vi "Read PublicEvents.vi"(8 "error in (no error)":errorcluster, 11 "SMOFacade in":refnum<class "SMOFacade.lvclass">) -> (0 "error out":errorcluster, 2 "SMO Base Events":T1, 3 "SMOFacade out":refnum<class "SMOFacade.lvclass">)   [LabVIEW 2013, in "SMOFacade.lvclass"]
uses:
  SMOFacade.lvclass
  SMO/Typedefs/Public Events.ctl
  SMO/Typedefs/SMOState --Enum.ctl
  SMO/Typedefs/Reserve State--Enum.ctl
  SMOFacade.lvclass/SMOFacade.ctl
  PublicEvents/PublicEvents.lvclass/PublicEvents.ctl
  PublicEvents/PublicEvents.lvclass
  SMO/SMO.lvclass
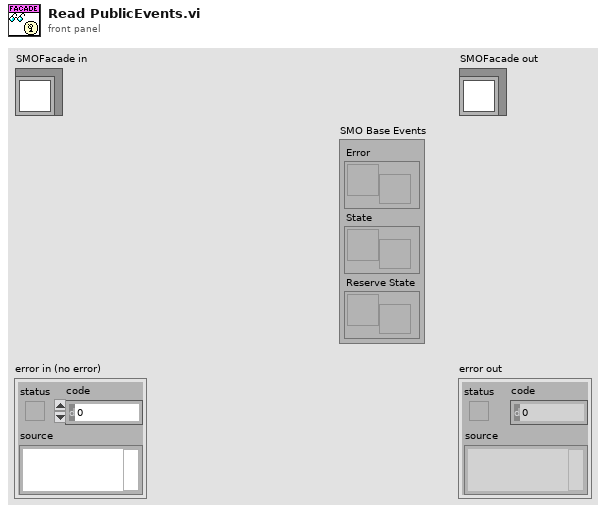
[diagram p1: front panel]
types:
  T1 = typedef "SMO.lvclass/Public Events.ctl" = cluster{"Error":refnum<user-event>, "State":refnum<user-event>, "Reserve State":refnum<user-event>}
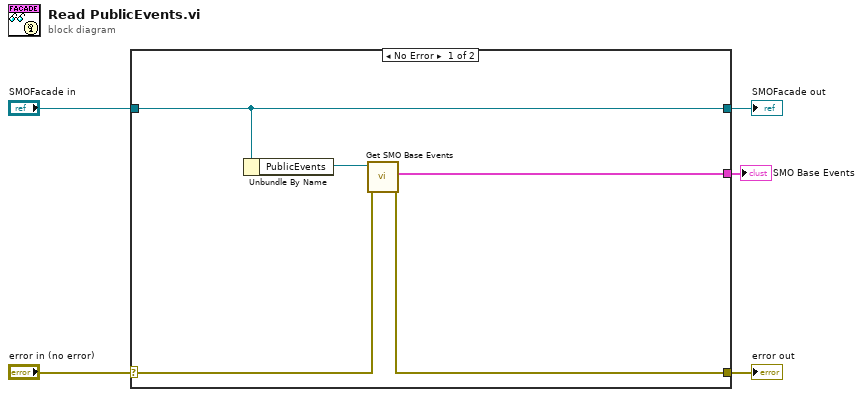
[diagram p0: block diagram]
diagram:
  n1 = case shown="No Error" "error in (no error)" {
    selector: "error in (no error)" -> [w8 w12]
    tunnel: [w7 w12] -> w4
    tunnel: [w10 w11] -> w2
    tunnel: "SMOFacade in" -> [w10 w11]
    tunnel: [w6 _] -> w1
    frame No Error {
      n2 = Unbundle By Name(w10) -> ("PublicEvents"=w9:refnum<class "PublicEvents.lvclass">)
      n3 = call "Get SMO Base Events.vi"("error in (no error)"=w8, "PublicEvents in"=w9) -> ("error out"=w7:errorcluster, "SMO Base Events"=w6:T1)  [unwired: 7 in, 1 out]
    }
    frame Error {
    }
  }
  "error out" <- w4
  "SMOFacade out" <- w2
  "SMO Base Events" <- w1
